vi "Engine-Throttle.vi"(8 "Error In":errorcluster, 11 "DSI Reference":refnum<class "DCM-DSI.lvclass">) -> (0 "Error Out":errorcluster, 3 "DSI Reference":refnum<class "DCM-DSI.lvclass">)   [LabVIEW 2016, in "DSI-RT.lvlib"]
uses:
  DSI-RT.lvlib
  Classes/DCM-DSI/DCM-DSI.lvclass
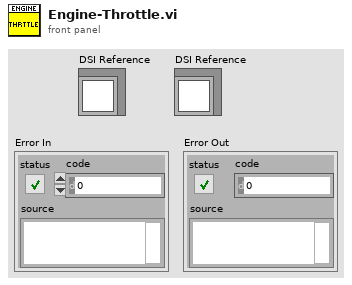
[diagram p1: front panel]
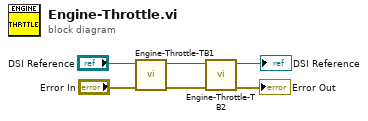
[diagram p0: block diagram]
diagram:
  n1 = call "Engine-Throttle-TB1.vi"("Error In"="Error In", "DSI Reference"="DSI Reference") -> ("Error Out"=w2:errorcluster, "DSI Reference"=w4:refnum<class "DCM-DSI.lvclass">)  [unwired: 8 in]
  n2 = call "Engine-Throttle-TB2.vi"("Error In"=w2, "DSI Reference"=w4) -> ("Error Out"=→"Error Out":errorcluster, "DSI Reference"=→"DSI Reference":refnum<class "DCM-DSI.lvclass">)  [unwired: 8 in]
